vi "ImageADC.vi"() -> ()   [LabVIEW 2012]
panel:
  out "reversed array 2":dbl[](array[numeric])
  out "Array 2":dbl[](array[numeric])
  out "Numeric 2":i32
  out "reversed array":i8[](array[numeric])
  out "output array 2":i8[][](array[numeric])
  out "x/y":dbl
  out "output array":i8[](array[numeric])
  out "0, 2":i16[][](array[numeric])
  in  "Array":dbl[](array[numeric])
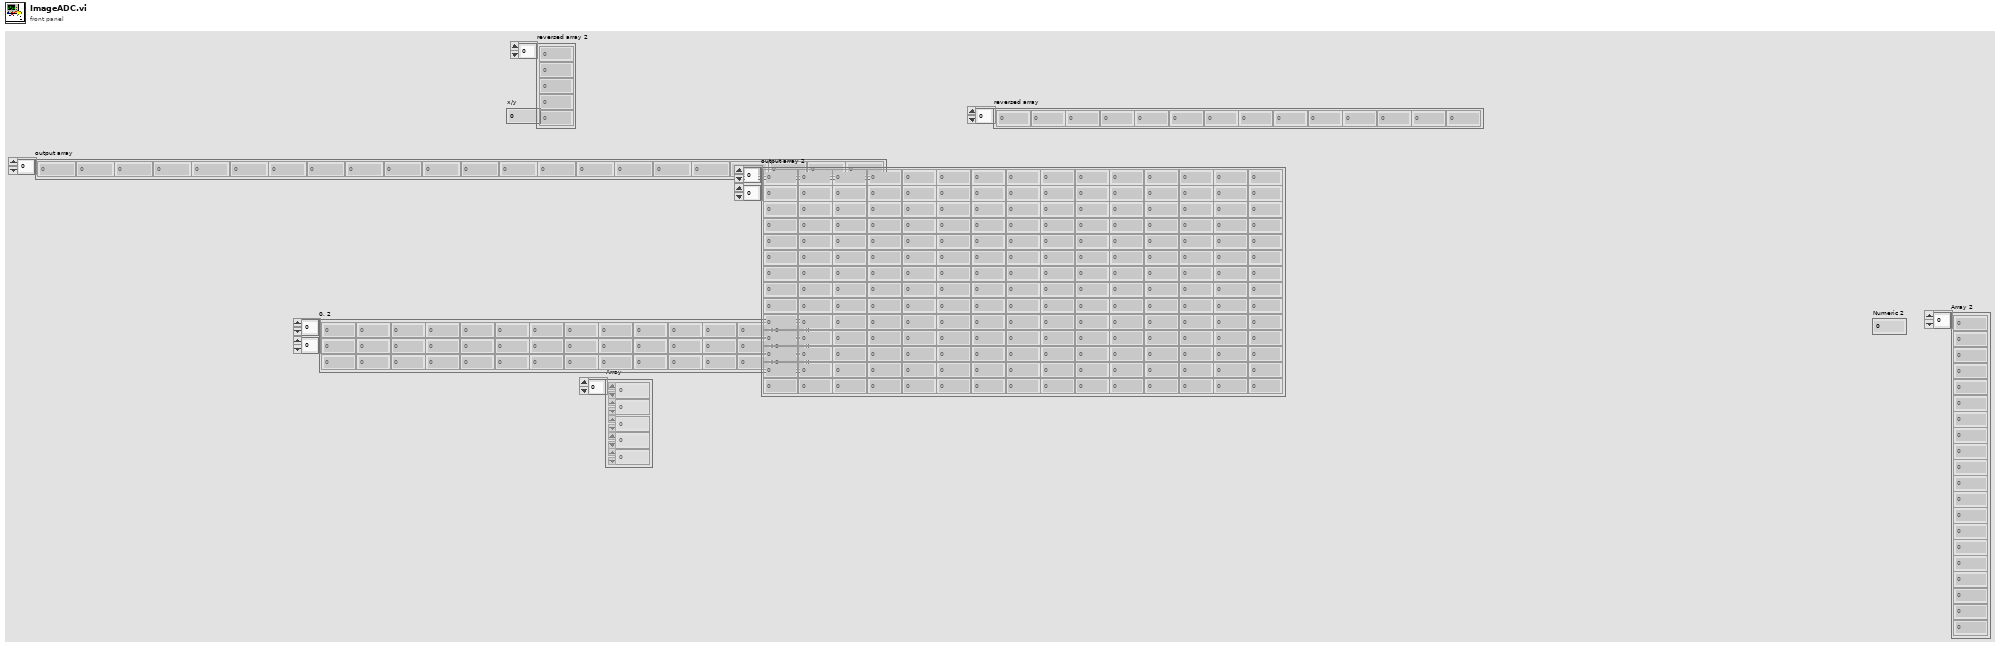
[diagram p1: front panel]
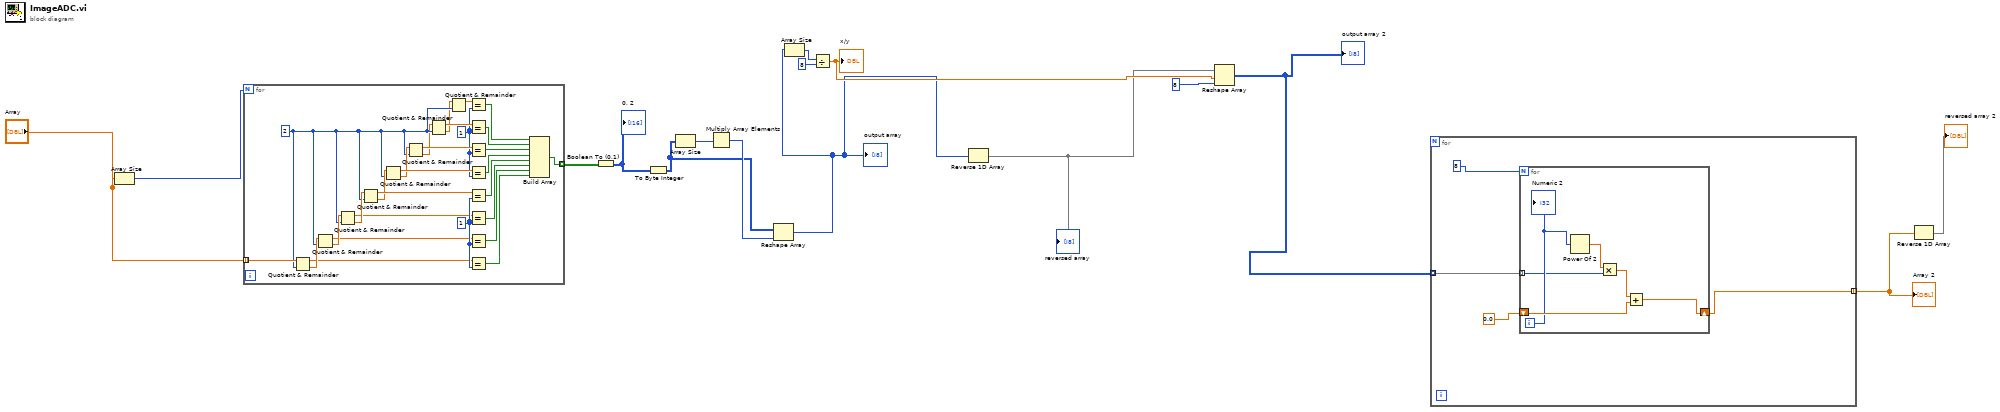
[diagram p0: block diagram]
diagram:
  n1 = Array Size(array="Array") -> (size(s)=w16:i32)
  n2 = for {
    N: w16 -> [_]
    tunnel: "Array" -> [w40] mode=indexing
    tunnel: [w17] -> w15 mode=indexing
    w31 = 1
    w28 = 2
    w41 = 1
    n3 = Quotient & Remainder(x=w40, y=w28) -> (x-y*floor(x/y)=w39:dbl, floor(x/y)=w42:dbl)
    n4 = Quotient & Remainder(x=w42, y=w28) -> (x-y*floor(x/y)=w38:dbl, floor(x/y)=w43:dbl)
    n5 = Quotient & Remainder(x=w43, y=w28) -> (x-y*floor(x/y)=w37:dbl, floor(x/y)=w44:dbl)
    n6 = Quotient & Remainder(x=w44, y=w28) -> (x-y*floor(x/y)=w36:dbl, floor(x/y)=w29:dbl)
    n7 = Quotient & Remainder(x=w29, y=w28) -> (x-y*floor(x/y)=w32:dbl, floor(x/y)=w30:dbl)
    n8 = Quotient & Remainder(x=w30, y=w28) -> (x-y*floor(x/y)=w33:dbl, floor(x/y)=w27:dbl)
    n9 = Quotient & Remainder(x=w27, y=w28) -> (x-y*floor(x/y)=w34:dbl, floor(x/y)=w26:dbl)
    n10 = Quotient & Remainder(x=w26, y=w28) -> (x-y*floor(x/y)=w35:dbl)  [unwired: 1 out]
    n11 = Equal?(x=w35, y=w31) -> (x = y?=w25:bool)
    n12 = Equal?(x=w34, y=w31) -> (x = y?=w24:bool)
    n13 = Equal?(x=w33, y=w31) -> (x = y?=w23:bool)
    n14 = Equal?(x=w32, y=w31) -> (x = y?=w22:bool)
    n15 = Equal?(x=w36, y=w41) -> (x = y?=w21:bool)
    n16 = Equal?(x=w37, y=w41) -> (x = y?=w20:bool)
    n17 = Equal?(x=w38, y=w41) -> (x = y?=w19:bool)
    n18 = Equal?(x=w39, y=w41) -> (x = y?=w18:bool)
    n19 = Build Array(w25, w24, w23, w22, w21, w20, w19, w18) -> (w17:bool[])
  }
  n20 = Boolean To (0,1)(Boolean=w15) -> (0, 1=w14:i16[][])
  "0, 2" <- w14
  n21 = To Byte Integer(number=w14) -> (8bit integer=w11:i8[][])
  n22 = Array Size(array=w11) -> (size(s)=w13:i32[])
  n23 = Multiply Array Elements(1:w13) -> (0:w12:i32)
  n24 = Reshape Array(w11, w12) -> (w5:i8[])
  "output array" <- w5
  n25 = Array Size(array=w5) -> (size(s)=w9:i32)
  n26 = Divide(x=w9, y=8) -> (x/y=w6:dbl)
  "x/y" <- w6
  n27 = Reverse 1D Array(array=w5) -> (reversed array=w4:i8[])
  "reversed array" <- w4
  n28 = Reshape Array(w4, w6, 8 ("dimension size")) -> (w3:i8[][])
  "output array 2" <- w3
  n29 = for {
    tunnel: [w46] -> w2 mode=indexing
    tunnel: w3 -> [w45] mode=indexing
    n30 = for {
      N: 8 -> [_]
      shift-right: [w52] -> w46
      shift-left: 0.0 -> [w53]
      tunnel: w45 -> [w49] mode=indexing
      i -> [w51]
      n31 = Power Of 2(x=w51) -> (2^x=w50:dbl)
      n32 = Multiply(x=w50, y=w49) -> (x*y=w54:dbl)
      n33 = Add(x=w54, y=w53) -> (x+y=w52:dbl)
      "Numeric 2" <- w51
    }
  }
  "Array 2" <- w2
  n34 = Reverse 1D Array(array=w2) -> (reversed array=→"reversed array 2":dbl[])
